vi "sort index for 1D array.vi"(2 "descending/ascending":bool, 3 "Array in":dbl[](array[numeric])) -> (0 "index":i32[](array[numeric]), 1 "sorted arrray":dbl[](array[numeric]))   [LabVIEW 2018]
panel:
  # "入力をソートしつつソート順の情報を取得する"
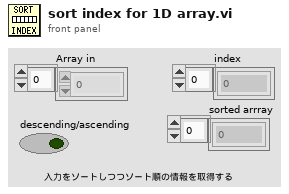
[diagram p1: front panel]
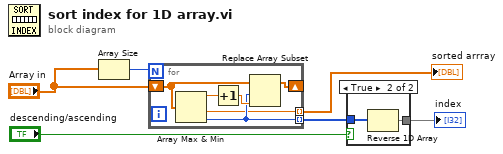
[diagram p0: block diagram]
diagram:
  n1 = Array Size(array="Array in") -> (size(s)=w3:i32)
  n2 = for {
    N: w3 -> [_]
    shift-right: [w9] -> _
    shift-left: "Array in" -> [w12]
    tunnel: [w8] -> w5 mode=indexing
    tunnel: [w7] -> w1 mode=indexing
    n3 = Array Max & Min(array=w12) -> (max value=w11:dbl, min value=w7:dbl, min index (indices)=w8:i32)  [unwired: 1 out]
    n4 = Increment(x=w11) -> (x+1=w10:dbl)
    n5 = Replace Array Subset(array=w12, new element=w10, index=w8) -> (w9:dbl[])
  }
  "sorted arrray" <- w1
  n6 = case shown="True" "descending/ascending" {
    tunnel: w5 -> [w13 w15]
    tunnel: [w13 w14] -> w6
    frame False {
    }
    frame True {
      n7 = Reverse 1D Array(array=w15) -> (reversed array=w14:i32[])
    }
  }
  "index" <- w6
